vi "Insert purchased_items.vi"(8 "Error In":errorcluster, 11 "Purchased_Items":T1 {"NumberOfUnits" format="%#.3g"}) -> (0 "Error Out":errorcluster, 3 "Output Data":string[][](array[string]))   [LabVIEW 2018, in "Database.lvlib"]
uses:
  Database.lvlib
  Purchased_Items--cluster.ctl
panel:
  out "Query [Debug]":string
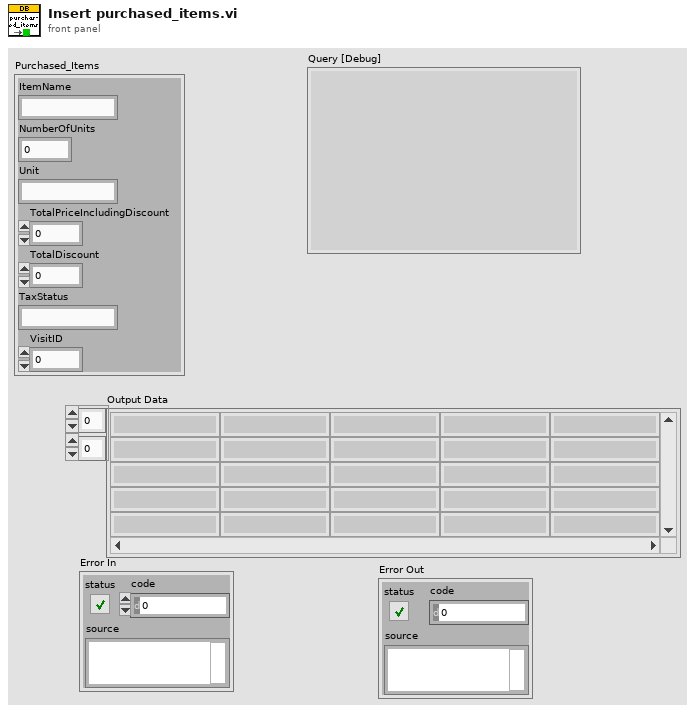
[diagram p1: front panel]
types:
  T1 = typedef "Database.lvlib/Purchased_Items--cluster.ctl" = cluster{"ItemName":string, "NumberOfUnits":dbl, "Unit":string, "TotalPriceIncludingDiscount":dbl, "TotalDiscount":dbl, "TaxStatus":string, "VisitID":i32}
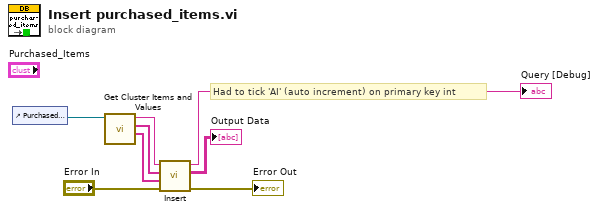
[diagram p0: block diagram]
diagram:
  # "Had to tick 'AI' (auto increment) on primary key int"
  n1 = control-ref of="Purchased_Items"() -> (w1:refnum<vi>)
  n2 = call "Get Cluster Items and Values.vi"("Generic Cluster Reference"=w1) -> ("String Values"=w7:string[], "Column"=w8:string[], "Table"=w6:string)  [unwired: 7 in, 1 out]
  n3 = call "Insert.vi"("error in (no error)"="Error In", "String Values"=w7, "Columns"=w8, "Table"=w6) -> ("error out"=→"Error Out":errorcluster, "Output Data"=→"Output Data":string[][], "Query [Debug]"=→"Query [Debug]":string)  [unwired: 5 in]
